vi "Configure Math.vi"(0 "VISA resource name":refnum<visa-resource-name>, 1 "Gain Coefficient (1)":dbl=1.0, 2 "Offset (0)":dbl, 5 "Enable Math (T: Enable)":bool=TRUE, 7 "Operation (0: Statistics)":u16(ring) items=["Statistics", "Scaling"], 9 "Enable Internal Result Storage (T: Enable)":bool=TRUE, 11 "error in (no error)":errorcluster) -> (4 "VISA resource name out":refnum<visa-resource-name>, 15 "error out":errorcluster)   [LabVIEW 2021, in "Agilent 34420.lvlib"]
doc: "Configures the math operation settings of the instrument."
uses:
  <instrlib>/Agilent 34420/Agilent 34420.lvlib
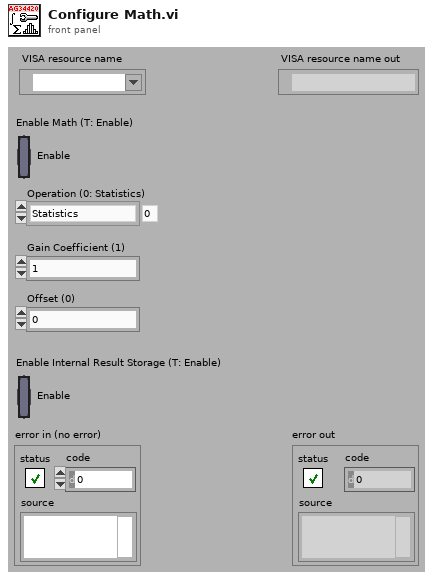
[diagram p1: front panel]
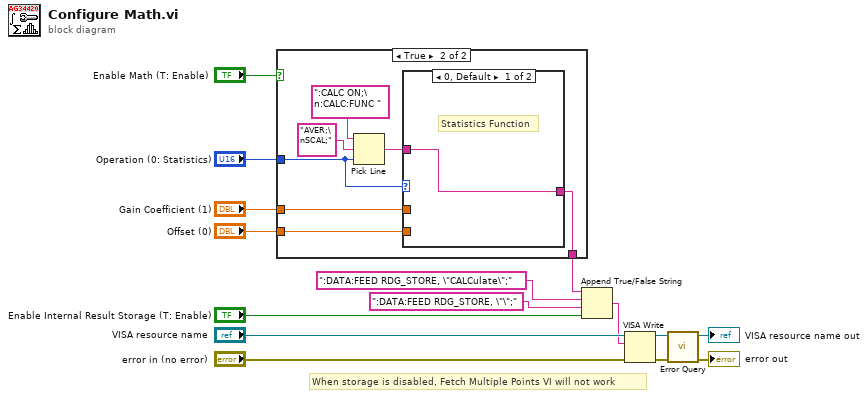
[diagram p0: block diagram]
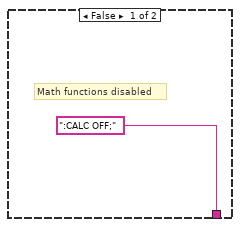
[diagram p2: hidden frame]
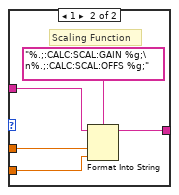
[diagram p3: hidden frame]
diagram:
  # "When storage is disabled, Fetch Multiple Points VI will not work"
  n1 = case shown="True" "Enable Math (T: Enable)" {
    tunnel: "Operation (0: Statistics)" -> [_ w21]
    tunnel: "Gain Coefficient (1)" -> [_ w19]
    tunnel: "Offset (0)" -> [_ w18]
    tunnel: [":CALC OFF;" ("output string") w17] -> w4
    frame False {
      # "Math functions disabled"
    }
    frame True {
      n2 = Pick Line(string ("")=":CALC ON;\n:CALC:FUNC ", multi-line string="AVER;\nSCAL;", line index=w21) -> (output string=w20:string)
      n3 = case shown="0, Default" w21 {
        tunnel: w20 -> [w24 w29]
        tunnel: w19 -> [_ w28]
        tunnel: w18 -> [_ w27]
        tunnel: [w24 w25] -> w17
        frame 0, Default {
          # "Statistics Function"
        }
        frame 1 {
          # "Scaling Function"
          n4 = Format Into String(format string="%.;:CALC:SCAL:GAIN %g;\n%.;:CALC:SCAL:OFFS %g;", initial string=w29, w28, w27) -> (resulting string=w25:string)  [unwired: 1 in, 1 out]
        }
      }
    }
  }
  n5 = Append True/False String(1:"Enable Internal Result Storage (T: Enable)", 2:":DATA:FEED RDG_STORE, \"\";" ("false string"), 3:":DATA:FEED RDG_STORE, \"CALCulate\";" ("true string"), 4:w4) -> (0:w5:string)
  n6 = VISA Write(VISA resource name="VISA resource name", write buffer=w5, error in (no error)="error in (no error)") -> (VISA resource name out=w11:refnum<visa-resource-name>, error out=w10:errorcluster)  [unwired: 1 out]
  n7 = call <instrlib>:"Error Query.vi"("error in (no error)"=w10, "VISA resource name"=w11) -> ("error out"=→"error out":errorcluster, "VISA resource name out"=→"VISA resource name out":refnum<visa-resource-name>)  [unwired: 6 in, 2 out]
